vi "(Sub) Disable Manager.vi"(1 "State":enum16{"Init", "Run", "Stop"}(ring), 2 "Run Butten":T1(ring), 5 "Run":refnum<vi>, 7 "Stop":refnum<vi>, 9 "Quick Stop":refnum<vi>, 11 "error in (no error)":errorcluster caption="에러 입력(에러 없음)") -> (15 "error out":errorcluster caption="에러 출력")   [LabVIEW 2017]
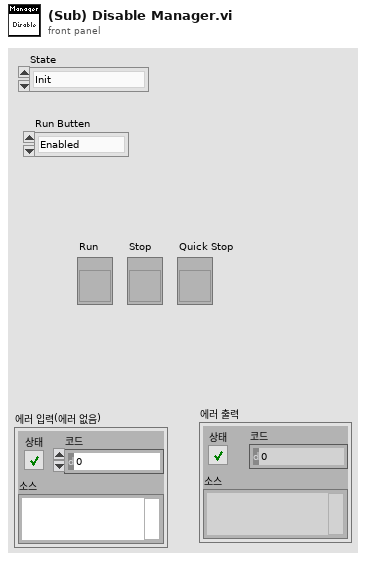
[diagram p1: front panel]
types:
  T1 = enum8{"Enabled", "Disabled", "Disabled and Grayed Out"}
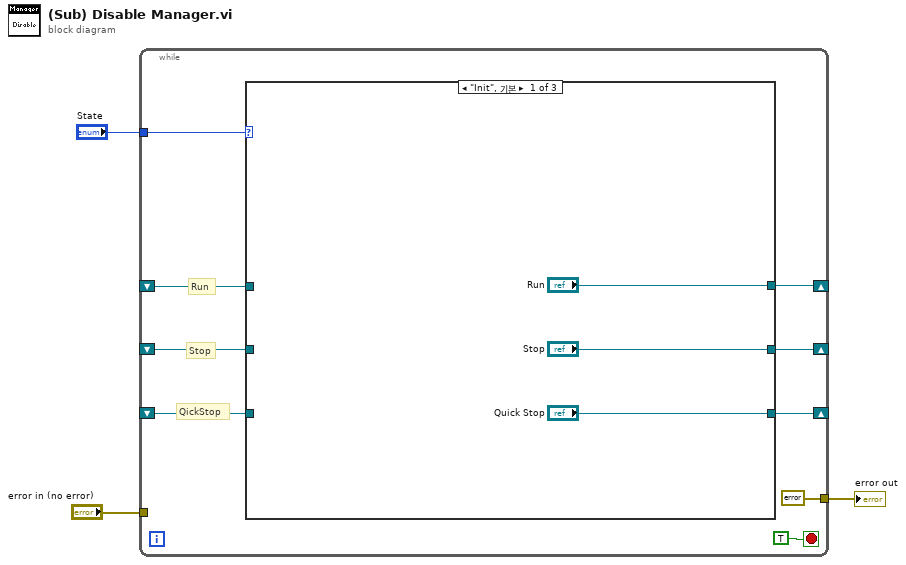
[diagram p0: block diagram]
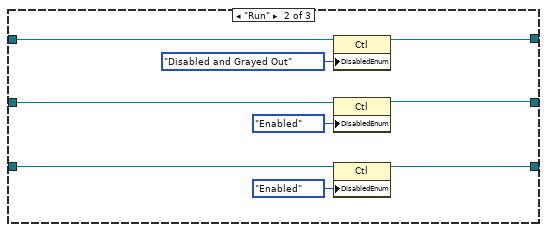
[diagram p2: hidden frame]
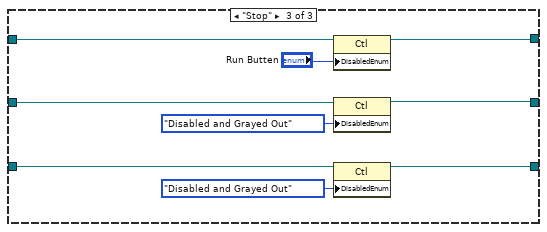
[diagram p3: hidden frame]
diagram:
  n1 = while {
    tunnel: "State" -> [w11]
    shift-right: [w10] -> _
    shift-left: _ -> [w7]
    shift-right: [w9] -> _
    shift-left: _ -> [w6]
    shift-right: [w8] -> _
    shift-left: _ -> [w5]
    tunnel: "error in (no error)" -> [_]
    tunnel: [errorcluster {"status"=FALSE, "code"=0, "source"=""} ("에러 상수")] -> w1
    stop <- TRUE stop-if-true
    # "QickStop"
    # "Stop"
    # "Run"
    n2 = case shown="\"Init\", 기본" w11 {
      tunnel: ["Run" w23 w32] -> w10
      tunnel: ["Stop" w21 w30] -> w9
      tunnel: ["Quick Stop" w19 w28] -> w8
      tunnel: w7 -> [_ w24 w33]
      tunnel: w6 -> [_ w22 w31]
      tunnel: w5 -> [_ w20 w29]
      frame "Init", Default {
      }
      frame "Run" {
        n3 = property class="Ctl"(reference=w24, "DisabledEnum"=T1."Disabled and Grayed Out" ("비활성화")) -> (reference out=w23:refnum<vi>)  [unwired: 1 in, 1 out]
        n4 = property class="Ctl"(reference=w22, "DisabledEnum"=T1."Enabled" ("비활성화")) -> (reference out=w21:refnum<vi>)  [unwired: 1 in, 1 out]
        n5 = property class="Ctl"(reference=w20, "DisabledEnum"=T1."Enabled" ("비활성화")) -> (reference out=w19:refnum<vi>)  [unwired: 1 in, 1 out]
      }
      frame "Stop" {
        n6 = property class="Ctl"(reference=w33, "DisabledEnum"="Run Butten") -> (reference out=w32:refnum<vi>)  [unwired: 1 in, 1 out]
        n7 = property class="Ctl"(reference=w31, "DisabledEnum"=T1."Disabled and Grayed Out" ("비활성화")) -> (reference out=w30:refnum<vi>)  [unwired: 1 in, 1 out]
        n8 = property class="Ctl"(reference=w29, "DisabledEnum"=T1."Disabled and Grayed Out" ("비활성화")) -> (reference out=w28:refnum<vi>)  [unwired: 1 in, 1 out]
      }
    }
  }
  "error out" <- w1
